vi "oa_Compare Time Stamps.vi"(1 "time stamp limit":timestamp, 2 "time stamp in":timestamp) -> (0 "greater than?":bool)   [LabVIEW 2017, in "SoundVib_OAUtility.lvlib"]
uses:
  <vilib>/addons/Sound and Vibration/Order Analysis/Utility/SoundVib_OAUtility.lvlib
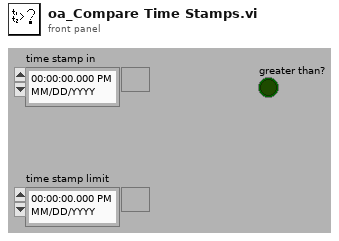
[diagram p1: front panel]
types:
  T1 = cluster{"second":i32, "minute":i32, "hour":i32, "day of month":i32, "month":i32, "year":i32, "day of week":i32, "day of year":i32, "is DST":i32}
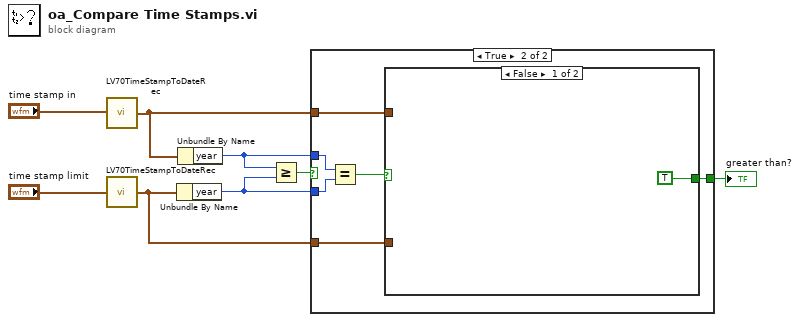
[diagram p0: block diagram]
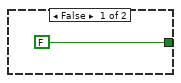
[diagram p2: hidden frame]
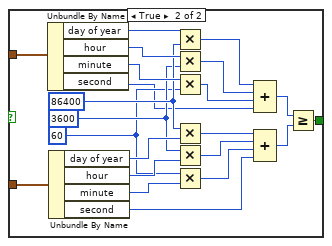
[diagram p3: hidden frame]
diagram:
  n1 = call <vilib>:"LV70TimeStampToDateRec.vi"("time stamp"="time stamp in") -> ("date time rec"=w7:T1)
  n2 = call <vilib>:"LV70TimeStampToDateRec.vi"("time stamp"="time stamp limit") -> ("date time rec"=w6:T1)
  n3 = Unbundle By Name(w6) -> ("year"=w1:i32)
  n4 = Unbundle By Name(w7) -> ("year"=w2:i32)
  n5 = Greater Or Equal?(x=w2, y=w1) -> (x >= y?=w8:bool)
  n6 = case shown="True" w8 {
    tunnel: [FALSE w13] -> w3
    tunnel: w7 -> [_ w14]
    tunnel: w6 -> [_ w15]
    tunnel: w2 -> [_ w12]
    tunnel: w1 -> [_ w11]
    frame False {
    }
    frame True {
      n7 = Equal?(x=w12, y=w11) -> (x = y?=w10:bool)
      n8 = case shown="False" w10 {
        tunnel: w15 -> [_ w38]
        tunnel: w14 -> [_ w37]
        tunnel: [TRUE w17] -> w13
        frame False {
        }
        frame True {
          w28 = 60
          w29 = 3600
          w30 = 86400
          n9 = Unbundle By Name(w37) -> ("day of year"=w31:i32, "hour"=w32:i32, "minute"=w33:i32, "second"=w24:i32)
          n10 = Unbundle By Name(w38) -> ("day of year"=w36:i32, "hour"=w35:i32, "minute"=w34:i32, "second"=w20:i32)
          n11 = Multiply(x=w31, y=w30) -> (x*y=w27:i32)
          n12 = Multiply(x=w32, y=w29) -> (x*y=w26:i32)
          n13 = Multiply(x=w33, y=w28) -> (x*y=w25:i32)
          n14 = Multiply(x=w30, y=w36) -> (x*y=w23:i32)
          n15 = Multiply(x=w29, y=w35) -> (x*y=w22:i32)
          n16 = Multiply(x=w28, y=w34) -> (x*y=w21:i32)
          n17 = Compound Arithmetic op=ADD(w27, w26, w25, w24) -> (w18:i32)
          n18 = Compound Arithmetic op=ADD(w23, w22, w21, w20) -> (w19:i32)
          n19 = Greater Or Equal?(x=w18, y=w19) -> (x >= y?=w17:bool)
        }
      }
    }
  }
  "greater than?" <- w3
